vi "Create.vi"(4 "Uncovered Node Count":i32, 5 "Fake Code Inspector in":refnum<class "Fake Code Inspector.lvclass">, 6 "Total Node Count":i32, 8 "error in (no error)":errorcluster, 9 "Uncovered Diagram Count":i32, 10 "Total Diagram Count":i32, 11 "VI Name":string) -> (0 "error out":errorcluster, 3 "Fake Code Inspector":refnum<class "Fake Code Inspector.lvclass">)   [LabVIEW 2017, in "Cobertura.Tests.lvlib" / "Fake Code Inspector.lvclass"]
uses:
  Fake Code Inspector.lvclass
  Fake Code Inspector.lvclass/Fake Code Inspector.ctl
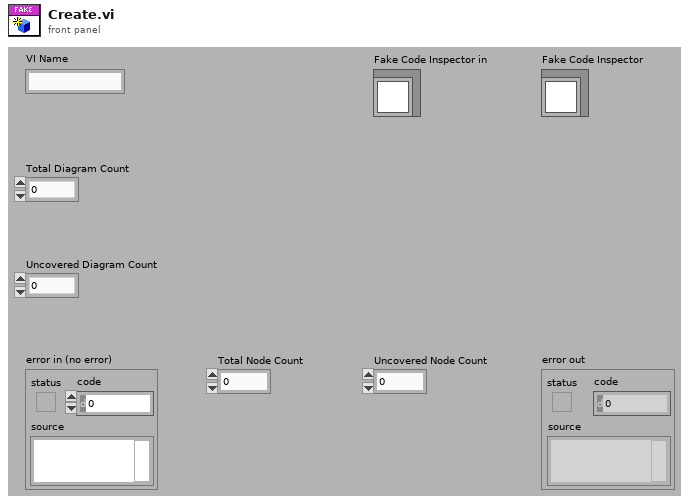
[diagram p1: front panel]
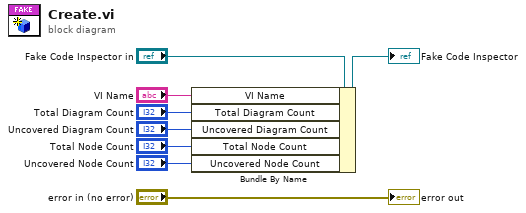
[diagram p0: block diagram]
diagram:
  n1 = Bundle By Name(cluster="Fake Code Inspector in", "VI Name"="VI Name", "Total Diagram Count"="Total Diagram Count", "Uncovered Diagram Count"="Uncovered Diagram Count", "Total Node Count"="Total Node Count", "Uncovered Node Count"="Uncovered Node Count") -> (→"Fake Code Inspector":refnum<class "Fake Code Inspector.lvclass">)
  "error out" <- "error in (no error)"
